vi "Delete_Table.vi"(6 "Auto?":bool, 8 "error in (no error)":errorcluster, 11 "Ref In":T1) -> (0 "error out":errorcluster)   [LabVIEW 2020]
uses:
  Controls/TD SQL.ctl
  <vilib>/addons/database/Connection.llb/Conn ObjectReference.ctl
  Controls/WIP_State.ctl
  MS SQL/MS_Global.vi
  <vilib>/addons/database/NI_Database_API.lvlib
  <vilib>/addons/database/Recordset.llb/Rec Save Format.ctl
  <vilib>/addons/database/Recordset.llb/Rec Destroy - Connection.vi
  <vilib>/addons/database/Recordset.llb/Rec Save Recordset To File (R).vi
  <vilib>/addons/database/Connection.llb/Conn Execute.vi
panel:
  out "Data Delete In Process...":dbl(slide) scale=0.0..1900.0
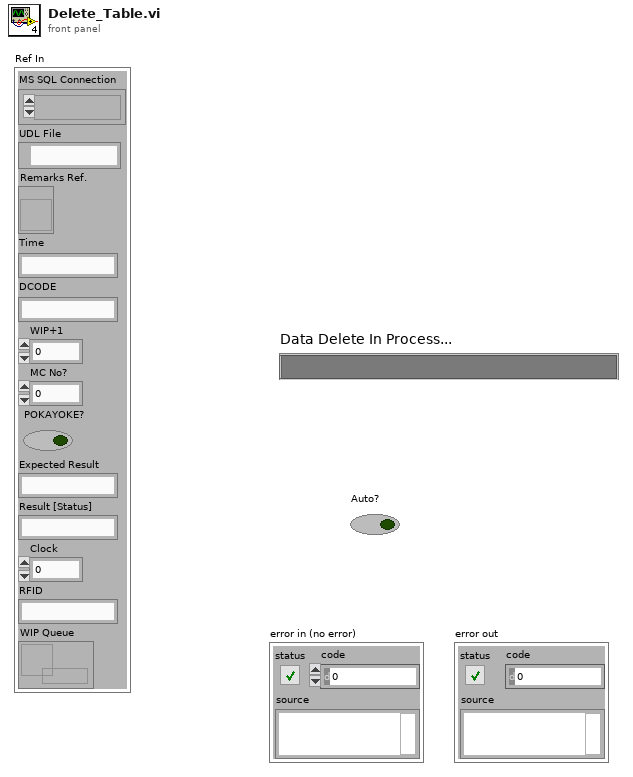
[diagram p1: front panel]
types:
  T1 = typedef "TD SQL.ctl" = cluster{"MS SQL Connection":T2, "UDL File":path, "Remarks Ref.":refnum<vi>, "Time":string, "DCODE":string, "WIP+1":i64, "MC No?":i32, "POKAYOKE?":bool, "Expected Result":string, "Result [Status]":string, "Clock":dbl, "RFID":string, "WIP Queue":refnum<queue>}
  T2 = typedef "NI_Database_API.lvlib/Conn ObjectReference.ctl" = refnum<k1>
  T3 = typedef "NI_Database_API.lvlib/Rec Save Format.ctl" = enum16{"ADTG", "XML"}
  T4 = typedef "NI_Database_API.lvlib/Rec ObjectReference.ctl" = refnum<k1>
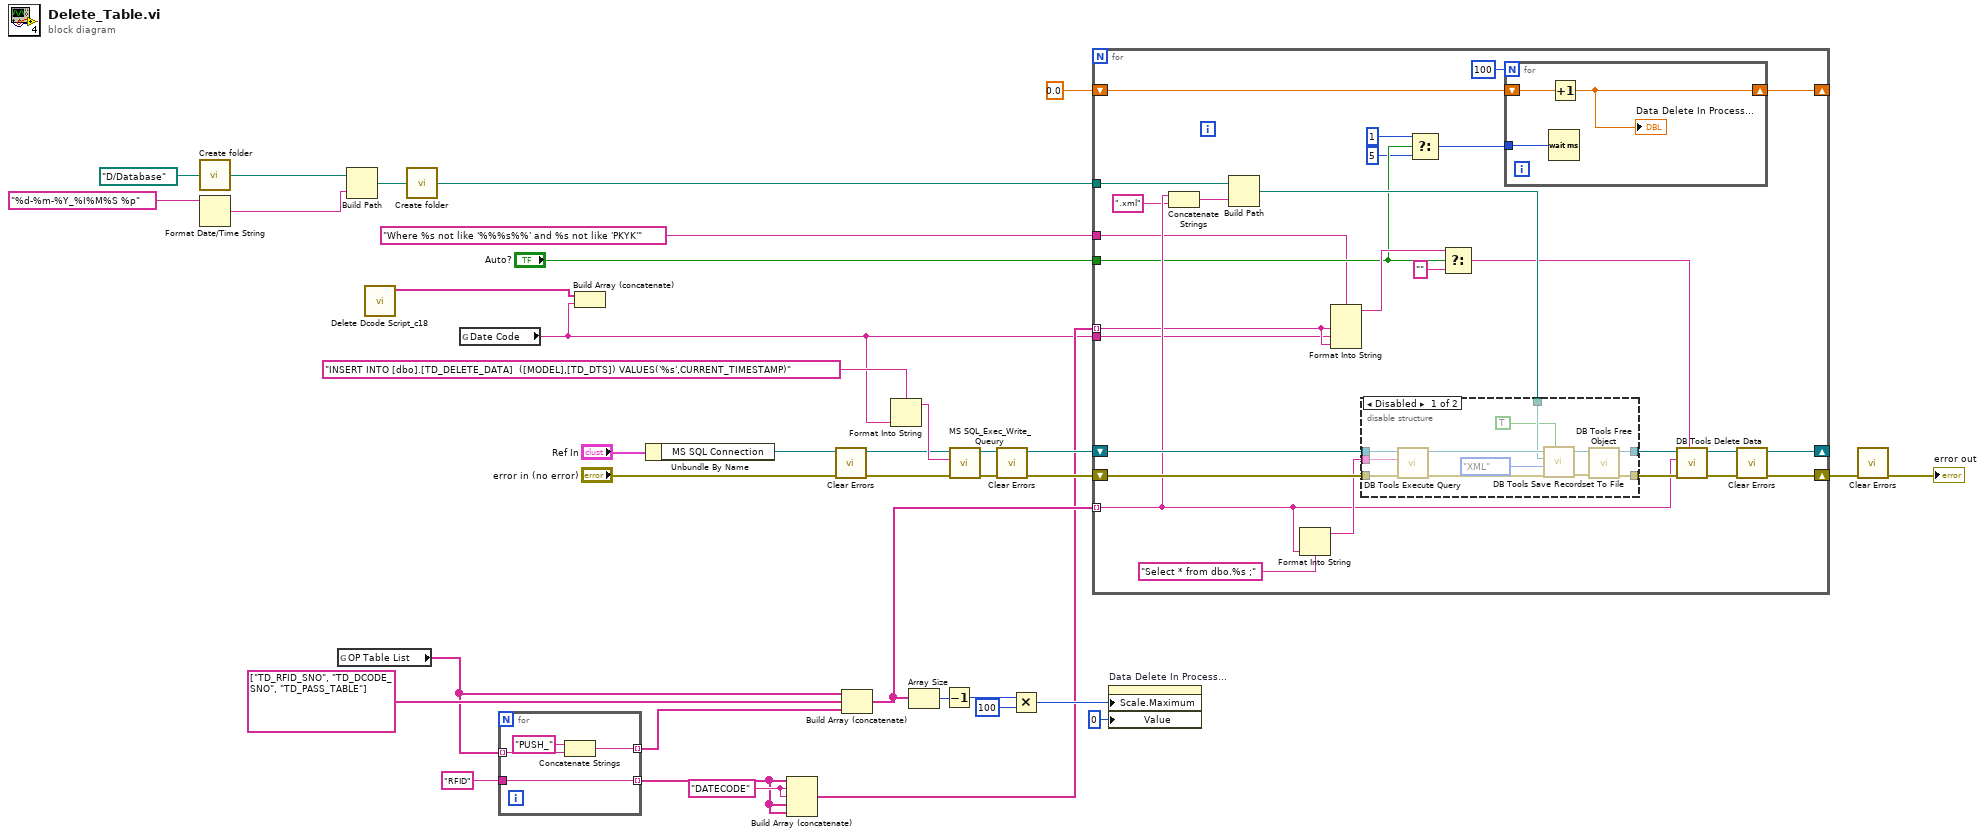
[diagram p0: block diagram]
diagram:
  w5 = "DATECODE" ("String")
  n1 = call <userlib>:"Create folder.vi"("Path In"=path "D:/Database") -> ("Path out"=w31:path)  [unwired: 14 in]
  n2 = Format Date/Time String(time format string (%c)="%d-%m-%Y_%I%M%S %p") -> (date/time string=w29:string)  [unwired: 2 in]
  n3 = global read "MS_Global.vi" "OP Table List"() -> (w8:string[])
  n4 = Build Path(base path=w31, name or relative path=w29) -> (appended path=w28:path)
  n5 = call "Delete Dcode Script_c18.vi"() -> ("Date Codes"=w2:string[])  [unwired: 11 in]
  n6 = call <userlib>:"Create folder.vi"("Path In"=w28) -> ("Path out"=w27:path)  [unwired: 14 in]
  n7 = global read "MS_Global.vi" "Date Code"() -> (w1:string)
  n8 = for {
    tunnel: w8 -> [w39] mode=indexing
    tunnel: [w37] -> w7 mode=indexing
    tunnel: [w36] -> w3 mode=indexing
    tunnel: "RFID" ("String") -> [w36]
    n9 = Concatenate Strings("PUSH_" ("string"), w39) -> (w37:string)
  }
  n10 = Build Array (concatenate)(w2, w1) -> ()  [unwired: 1 out]
  n11 = Unbundle By Name("Ref In") -> ("MS SQL Connection"=w15:T2)
  n12 = Build Array (concatenate)(w3, w5, w5, w3, w3) -> (w4:string[])
  n13 = call <vilib>:"Clear Errors.vi"("error in (no error)"="error in (no error)") -> ("error out"=w13:errorcluster)  [unwired: 5 in, 1 out]
  n14 = Build Array (concatenate)(w8, string[] ["TD_RFID_SNO", "TD_DCODE_SNO", "TD_PASS_TABLE"] ("tables"), w7) -> (w9:string[])
  n15 = Format Into String(format string="INSERT INTO [dbo].[TD_DELETE_DATA]  ([MODEL],[TD_DTS]) VALUES('%s',CURRENT_TIMESTAMP)" ("String"), w1) -> (resulting string=w16:string)  [unwired: 2 in, 1 out]
  n16 = Array Size(array=w9) -> (size(s)=w21:i32)
  n17 = Decrement(x=w21) -> (x-1=w25:i32)
  n18 = call "MS SQL_Exec_Write_Queury.vi"("error in (no error)"=w13, "Query"=w16, "Refnum in"=w15) -> ("error out"=w12:errorcluster, "Refnum out"=w14:T2)  [unwired: 7 in]
  n19 = call <vilib>:"Clear Errors.vi"("error in (no error)"=w12) -> ("error out"=w11:errorcluster)  [unwired: 5 in, 1 out]
  n20 = Multiply(x=w25, y=100) -> (x*y=w24:i32)
  n21 = for {
    tunnel: w9 -> [w57] mode=indexing
    shift-right: [w50] -> w34
    shift-left: w11 -> [w62]
    shift-right: [w65] -> _
    shift-left: w14 -> [w64]
    tunnel: w27 -> [w58]
    shift-right: [w52] -> _
    shift-left: 0.0 ("Delete In Process...") -> [w51]
    tunnel: w4 -> [w41] mode=indexing
    tunnel: "Auto?" -> [w46]
    tunnel: "Where %s not like '%%%s%%' and %s not like 'PKYK'" ("SQL query") -> [w42]
    tunnel: w1 -> [w40]
    n22 = Concatenate Strings(w57, ".xml" ("string")) -> (w55:string)
    n23 = Build Path(base path=w58, name or relative path=w55) -> (appended path=w54:path)
    n24 = Format Into String(format string="Select * from dbo.%s ;" ("SQL query"), w57) -> (resulting string=w59:string)  [unwired: 2 in, 1 out]
    n25 = Format Into String(format string=w42, w41, w40, w41) -> (resulting string=w49:string)  [unwired: 2 in, 1 out]
    n26 = disable-structure shown="Disabled" {
      disable-tunnel: w64 -> [w76 _]
      disable-tunnel: [w73 _] -> w63
      disable-tunnel: w62 -> [w72 _]
      disable-tunnel: [w71 _] -> w61
      disable-tunnel: w59 -> [w70 _]
      disable-tunnel: w54 -> [w69 _]
      frame Disabled {
        n27 = call-poly <vilib>:"DB Tools Execute Query.vi"("error in (no error)"=w72, "SQL query"=w70, "connection reference"=w76) -> ("error out"=w77:errorcluster, "recordset reference"=w78:T4)  [unwired: 5 in]
        n28 = call-poly <vilib>:"DB Tools Save Recordset To File.vi"("overwrite? (F)"=TRUE, "error in (no error)"=w77, "save format (XML)"=Rec_Save_Format."XML", "file name"=w69, "recordset reference"=w78) -> ("error out"=w75:errorcluster, "recordset reference out"=w74:T4)  [unwired: 3 in]
        n29 = call-poly <vilib>:"DB Tools Free Object.vi"("error in (no error)"=w75, "recordset reference"=w74) -> ("error out"=w71:errorcluster, "connection reference"=w73:T2)  [unwired: 8 in]
      }
      frame Enabled {
      }
    }
    n30 = Select(t=u32 1 ("milliseconds to wait"), s=w46, f=u32 5 ("milliseconds to wait")) -> (s? t:f=w43:u32)
    n31 = Select(t=w49, s=w46, f="") -> (s? t:f=w47:string)
    n32 = for {
      N: 100 -> [_]
      shift-right: [w80] -> w52
      shift-left: w51 -> [w81]
      tunnel: w43 -> [w79]
      n33 = Wait (ms)(milliseconds to wait=w79) -> ()  [unwired: 1 out]
      n34 = Increment(x=w81) -> (x+1=w80:dbl)
      "Data Delete In Process..." <- w80
    }
    n35 = call <vilib>:"DB Tools Delete Data.vi"("condition"=w47, "error in (no error)"=w61, "table"=w57, "connection reference"=w63) -> ("error out"=w66:errorcluster, "connection reference out"=w65:T2)  [unwired: 6 in]
    n36 = call <vilib>:"Clear Errors.vi"("error in (no error)"=w66) -> ("error out"=w50:errorcluster)  [unwired: 5 in, 1 out]
  }
  n37 = property on="Data Delete In Process..." class="Slide (strict)"("Scale.Maximum"=w24, "Value"=u8 0 ("Delete In Process...")) -> ()  [unwired: 2 in, 2 out]
  n38 = call <vilib>:"Clear Errors.vi"("error in (no error)"=w34) -> ("error out"=→"error out":errorcluster)  [unwired: 5 in, 1 out]
